vi "Kinesis - PDXC2 - Connect Move.vi"() -> ()   [LabVIEW 2013]
uses:
  C:/Users/zizhang/OneDrive - THORLABS Inc/Documents/4. SW Project/PDXC2/LabVIEW/Thorlabs.MotionControl.Controls.dll
  4. SW Project/PDXC2/LabVIEW/Thorlabs.MotionControl.Controls.dll
  C:/Users/zizhang/OneDrive - THORLABS Inc/Documents/4. SW Project/PDXC2/LabVIEW/Thorlabs.MotionControl.Benchtop.PiezoCLI.dll
  4. SW Project/PDXC2/LabVIEW/Thorlabs.MotionControl.Benchtop.PiezoCLI.dll
panel:
  in  "Tab Control":enum32{"Closed Loop", "Open Loop"}(tab)
  out "Current Position (nm)":i32
  in  "Target Position (nm)":i32
  out "Current Position (steps)":i32
  in  "Target Position (steps)":i32
  in  "SerialNumber":string
  in  "BenchtopPDXC2Control":refnum<k24>(container)
  # "Thorlabs Hardware: PDXC2 - Compact Single Stage ORIC Piezo Inertia Stage Controller\nhttps://www.thorlabs.com/thorproduct.cfm?partnumber=PDXC2\n\nDescription: This VI will enable you to communicate with PDXC2 series to control Piezo Inertia Stages. The VI will first connect and initialize the device, home the stage if the \"Closed Loop\" tab is enabled, and move the stage to a specified location.\n\nInstructions: \n1) Connect your device to your PC & power the device. ensuring your stage/actutator is connected prior to power the device. For full device setup, the device product manual can be found on our website.\n2) Enter the device serial number and the target position below.\n3) If the stage is equipped with encoders and the \"Closed Loop\" tab is enabled, ensure the device move path is clear for homing.\n4) Click 'Run' in the LabVIEW Toolbar which will attempt a connection. And a home command will be sent when the \"Closed Loop\" tab is enabled.\n5) Await for device to be available, the stage will move to the target position."
  # "Only for PDX Series Stages"
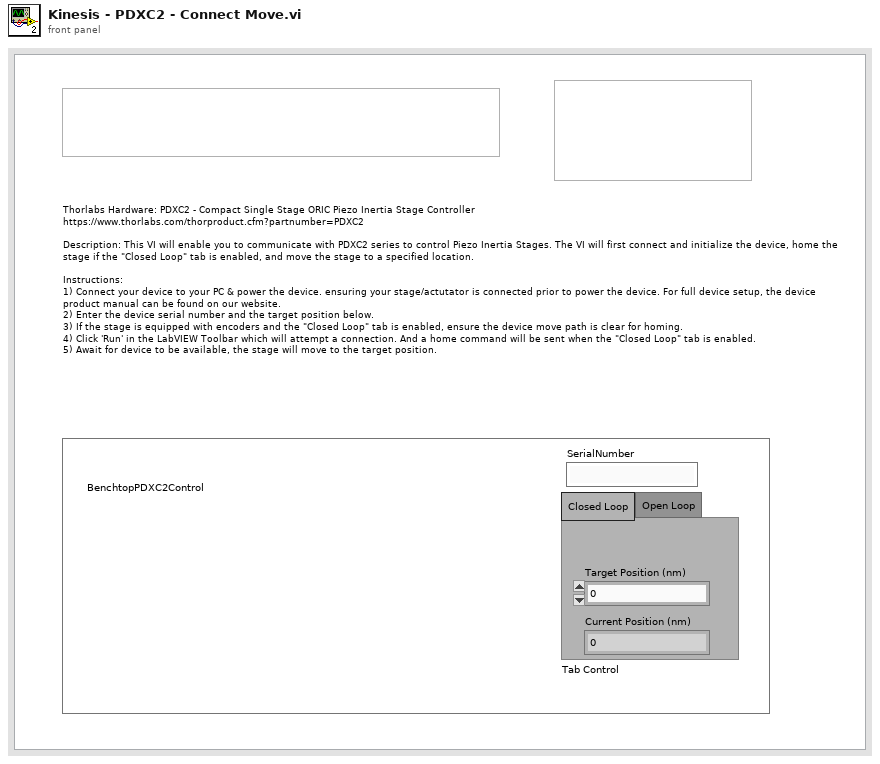
[diagram p1: front panel]
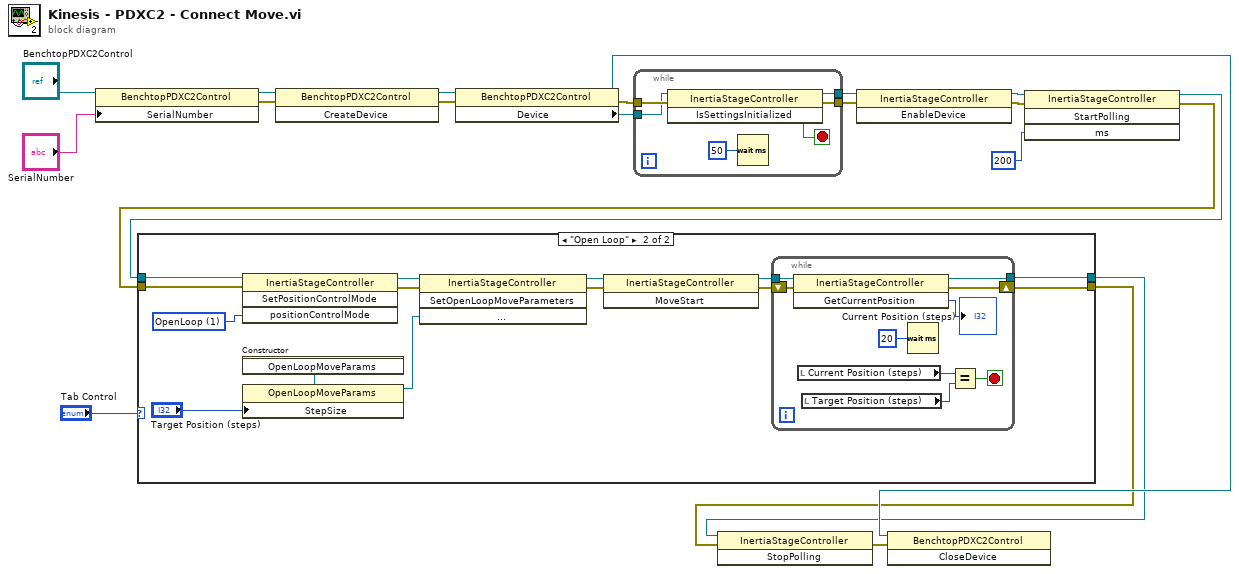
[diagram p0: block diagram]
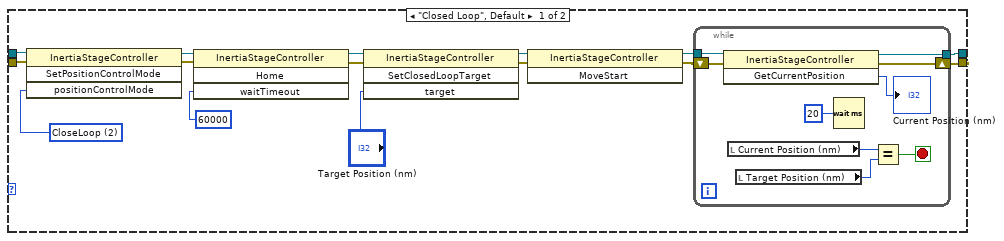
[diagram p2: hidden frame]
diagram:
  n1 = property class="BenchtopPDXC2Control"(reference="BenchtopPDXC2Control", "SerialNumber"="SerialNumber") -> (reference out=w18:refnum<k24>, error out=w17:errorcluster)  [unwired: 1 in]
  n2 = invoke class="BenchtopPDXC2Control" method="CreateDevice"(reference=w18, error in=w17) -> (reference out=w16:refnum<k24>, error out=w15:errorcluster)  [unwired: 1 in, 1 out]
  n3 = property class="BenchtopPDXC2Control"(reference=w16, error in=w15) -> (reference out=w13:refnum<k24>, error out=w14:errorcluster, "Device"=w3:refnum<k24>)
  n4 = while {
    tunnel: [w25] -> w12
    tunnel: w14 -> [w22]
    tunnel: [w23] -> w11
    tunnel: w3 -> [w21]
    stop <- w26 stop-if-true
    n5 = invoke class="InertiaStageController" method="IsSettingsInitialized"(reference=w21, error in=w22) -> (reference out=w25:refnum<k24>, error out=w23:errorcluster, "IsSettingsInitialized"=w26:bool)  [unwired: 1 in]
    n6 = Wait (ms)(milliseconds to wait=u32 50) -> ()  [unwired: 1 out]
  }
  n7 = invoke class="InertiaStageController" method="EnableDevice"(reference=w12, error in=w11) -> (reference out=w9:refnum<k24>, error out=w5:errorcluster)  [unwired: 1 in, 1 out]
  n8 = invoke class="InertiaStageController" method="StartPolling"(reference=w9, error in=w5, "ms"=200) -> (reference out=w8:refnum<k24>, error out=w4:errorcluster)  [unwired: 1 in, 2 out]
  n9 = case shown="\"Open Loop\"" "Tab Control" {
    tunnel: w8 -> [w32 w63]
    tunnel: [w38 w58] -> w7
    tunnel: [w37 w57] -> w6
    tunnel: w4 -> [w31 w56]
    frame "Closed Loop", Default {
      w41 = 2 items=["OpenLoop"=1, "CloseLoop"=2, "OpenLoopSmooth"=3, "CloseLoopSmooth"=4] ("positionControlMode")
      n10 = invoke class="InertiaStageController" method="SetPositionControlMode"(reference=w32, error in=w31, "positionControlMode"=w41) -> (reference out=w29:refnum<k24>, error out=w30:errorcluster)  [unwired: 1 in, 2 out]
      n11 = invoke class="InertiaStageController" method="Home"(reference=w29, error in=w30, "waitTimeout"=60000) -> (reference out=w28:refnum<k24>, error out=w27:errorcluster)  [unwired: 1 in, 2 out]
      n12 = invoke class="InertiaStageController" method="SetClosedLoopTarget"(reference=w28, error in=w27, "target"="Target Position (nm)") -> (reference out=w40:refnum<k24>, error out=w36:errorcluster)  [unwired: 1 in, 2 out]
      n13 = invoke class="InertiaStageController" method="MoveStart"(reference=w40, error in=w36) -> (reference out=w39:refnum<k24>, error out=w35:errorcluster)  [unwired: 1 in, 1 out]
      n14 = while {
        tunnel: [w46] -> w38
        shift-right: [w49] -> w37
        shift-left: w35 -> [w47]
        tunnel: w39 -> [w45]
        stop <- w50 stop-if-true
        n15 = invoke class="InertiaStageController" method="GetCurrentPosition"(reference=w45, error in=w47) -> (reference out=w46:refnum<k24>, error out=w49:errorcluster, "GetCurrentPosition"=→"Current Position (nm)":i32)  [unwired: 1 in]
        n16 = local read "Current Position (nm)"() -> (w44:i32)
        n17 = local read "Target Position (nm)"() -> (w43:i32)
        n18 = Wait (ms)(milliseconds to wait=u32 20) -> ()  [unwired: 1 out]
        n19 = Equal?(x=w44, y=w43) -> (x = y?=w50:bool)
      }
    }
    frame "Open Loop" {
      w64 = 1 items=["OpenLoop"=1, "CloseLoop"=2, "OpenLoopSmooth"=3, "CloseLoopSmooth"=4] ("positionControlMode")
      n20 = invoke class="InertiaStageController" method="SetPositionControlMode"(reference=w63, error in=w56, "positionControlMode"=w64) -> (reference out=w62:refnum<k24>, error out=w55:errorcluster)  [unwired: 1 in, 2 out]
      n21 = constructor class="OpenLoopMoveParams"() -> (reference out=w52:refnum<k24>)  [unwired: 3 in, 2 out]
      n22 = property class="OpenLoopMoveParams"(reference=w52, "StepSize"="Target Position (steps)") -> (reference out=w61:refnum<k24>)  [unwired: 1 in, 1 out]
      n23 = invoke class="InertiaStageController" method="SetOpenLoopMoveParameters"(reference=w62, error in=w55, "parameters"=w61) -> (reference out=w60:refnum<k24>, error out=w54:errorcluster)  [unwired: 1 in, 2 out]
      n24 = invoke class="InertiaStageController" method="MoveStart"(reference=w60, error in=w54) -> (reference out=w59:refnum<k24>, error out=w53:errorcluster)  [unwired: 1 in, 1 out]
      n25 = while {
        tunnel: [w67] -> w58
        shift-right: [w72] -> w57
        shift-left: w53 -> [w68]
        tunnel: w59 -> [w66]
        stop <- w73 stop-if-true
        n26 = invoke class="InertiaStageController" method="GetCurrentPosition"(reference=w66, error in=w68) -> (reference out=w67:refnum<k24>, error out=w72:errorcluster, "GetCurrentPosition"=→"Current Position (steps)":i32)  [unwired: 1 in]
        n27 = local read "Current Position (steps)"() -> (w71:i32)
        n28 = local read "Target Position (steps)"() -> (w70:i32)
        n29 = Wait (ms)(milliseconds to wait=u32 20) -> ()  [unwired: 1 out]
        n30 = Equal?(x=w71, y=w70) -> (x = y?=w73:bool)
      }
    }
  }
  n31 = invoke class="InertiaStageController" method="StopPolling"(reference=w7, error in=w6) -> (error out=w1:errorcluster)  [unwired: 1 in, 2 out]
  n32 = invoke class="BenchtopPDXC2Control" method="CloseDevice"(reference=w13, error in=w1) -> ()  [unwired: 1 in, 3 out]
